vi "LCD Control Panel (No Objects).vi"(8 "error in (no error)":errorcluster) -> (0 "error out":errorcluster)   [LabVIEW 2012]
uses:
  <vilib>/DAQmx/write.llb/DAQmx Write (Analog DBL 1Chan 1Samp).vi
  <vilib>/DAQmx/create/channels.llb/DAQmx Create Channel (AO-Voltage-Basic).vi
  <vilib>/DAQmx/miscellaneous.llb/DAQmx Fill In Error Info.vi
panel:
  out "done":bool
  in  "Analog \nOutput \nSync":bool
  in  "Alternate":bool
  in  "Frequency":dbl=0.01 min=0.01 max=6.0
  out "?":bool
  out "?":bool
  in  "Retardance 2":dbl
  in  "Retardance 1":dbl
  in  "stop":bool
  out "error":bool caption="Error"
  in  "Check for Instrument":bool
  out "Current Retardance":dbl[unit] caption="Retardance"
  out "Ready":bool
  in  "waveoptions":T1(radio) caption="Wave Options"
  in  "Wavelength":dbl[unit]=7.81e-07
  out "Title":string="LCD Retarder Control Program"
  in  "Zero":bool
  in  "Set\nRetardance":bool
  in  "Goto Retardance":dbl[unit]
  in  "Exit":bool
  # "and"
  # "at"
  # "Hz"
  # "between"
  # "Note from John: Analog Output #0 will toggle from 0 to 1 V in synch with this."
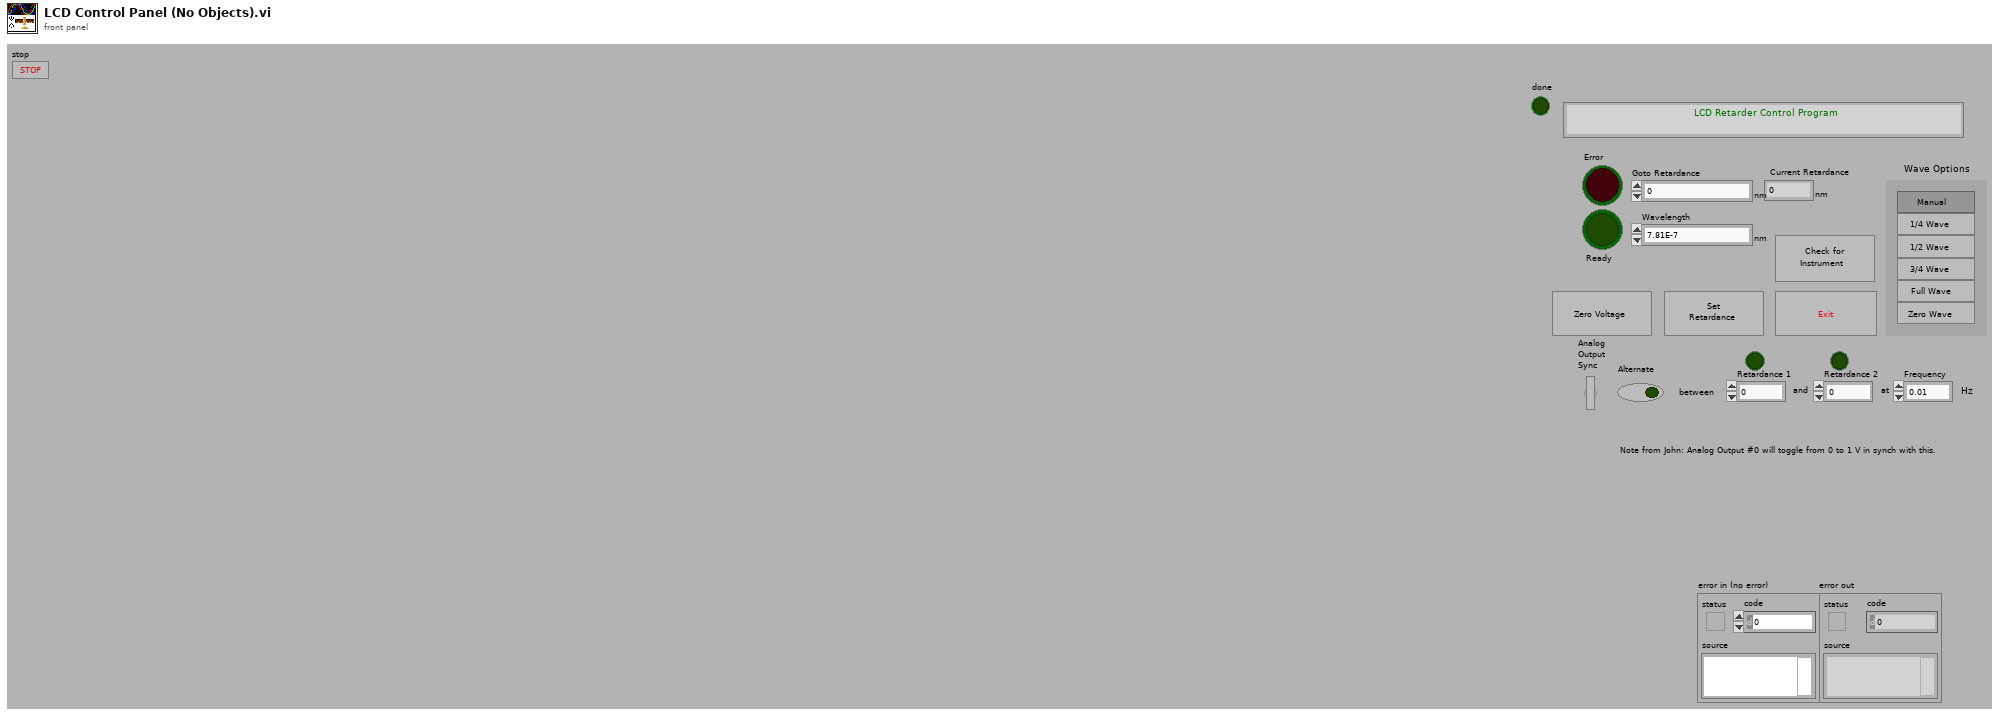
[diagram p1: front panel]
types:
  T1 = enum32{"Manual", "1/4 Wave", "1/2 Wave", "3/4 Wave", "Full Wave", "Zero Wave"}
  T2 = cluster{"Retardance":dbl[unit], "LCD Handle":cluster{"Device Handle":u32, "Pipe 0 Handle":u32, "Pipe 1 Handle":u32}, "All open LCD Handles":cluster{"Device Handle":u32, "Pipe 0 Handle":u32, "Pipe 1 Handle":u32}[], "FW Version":dbl}
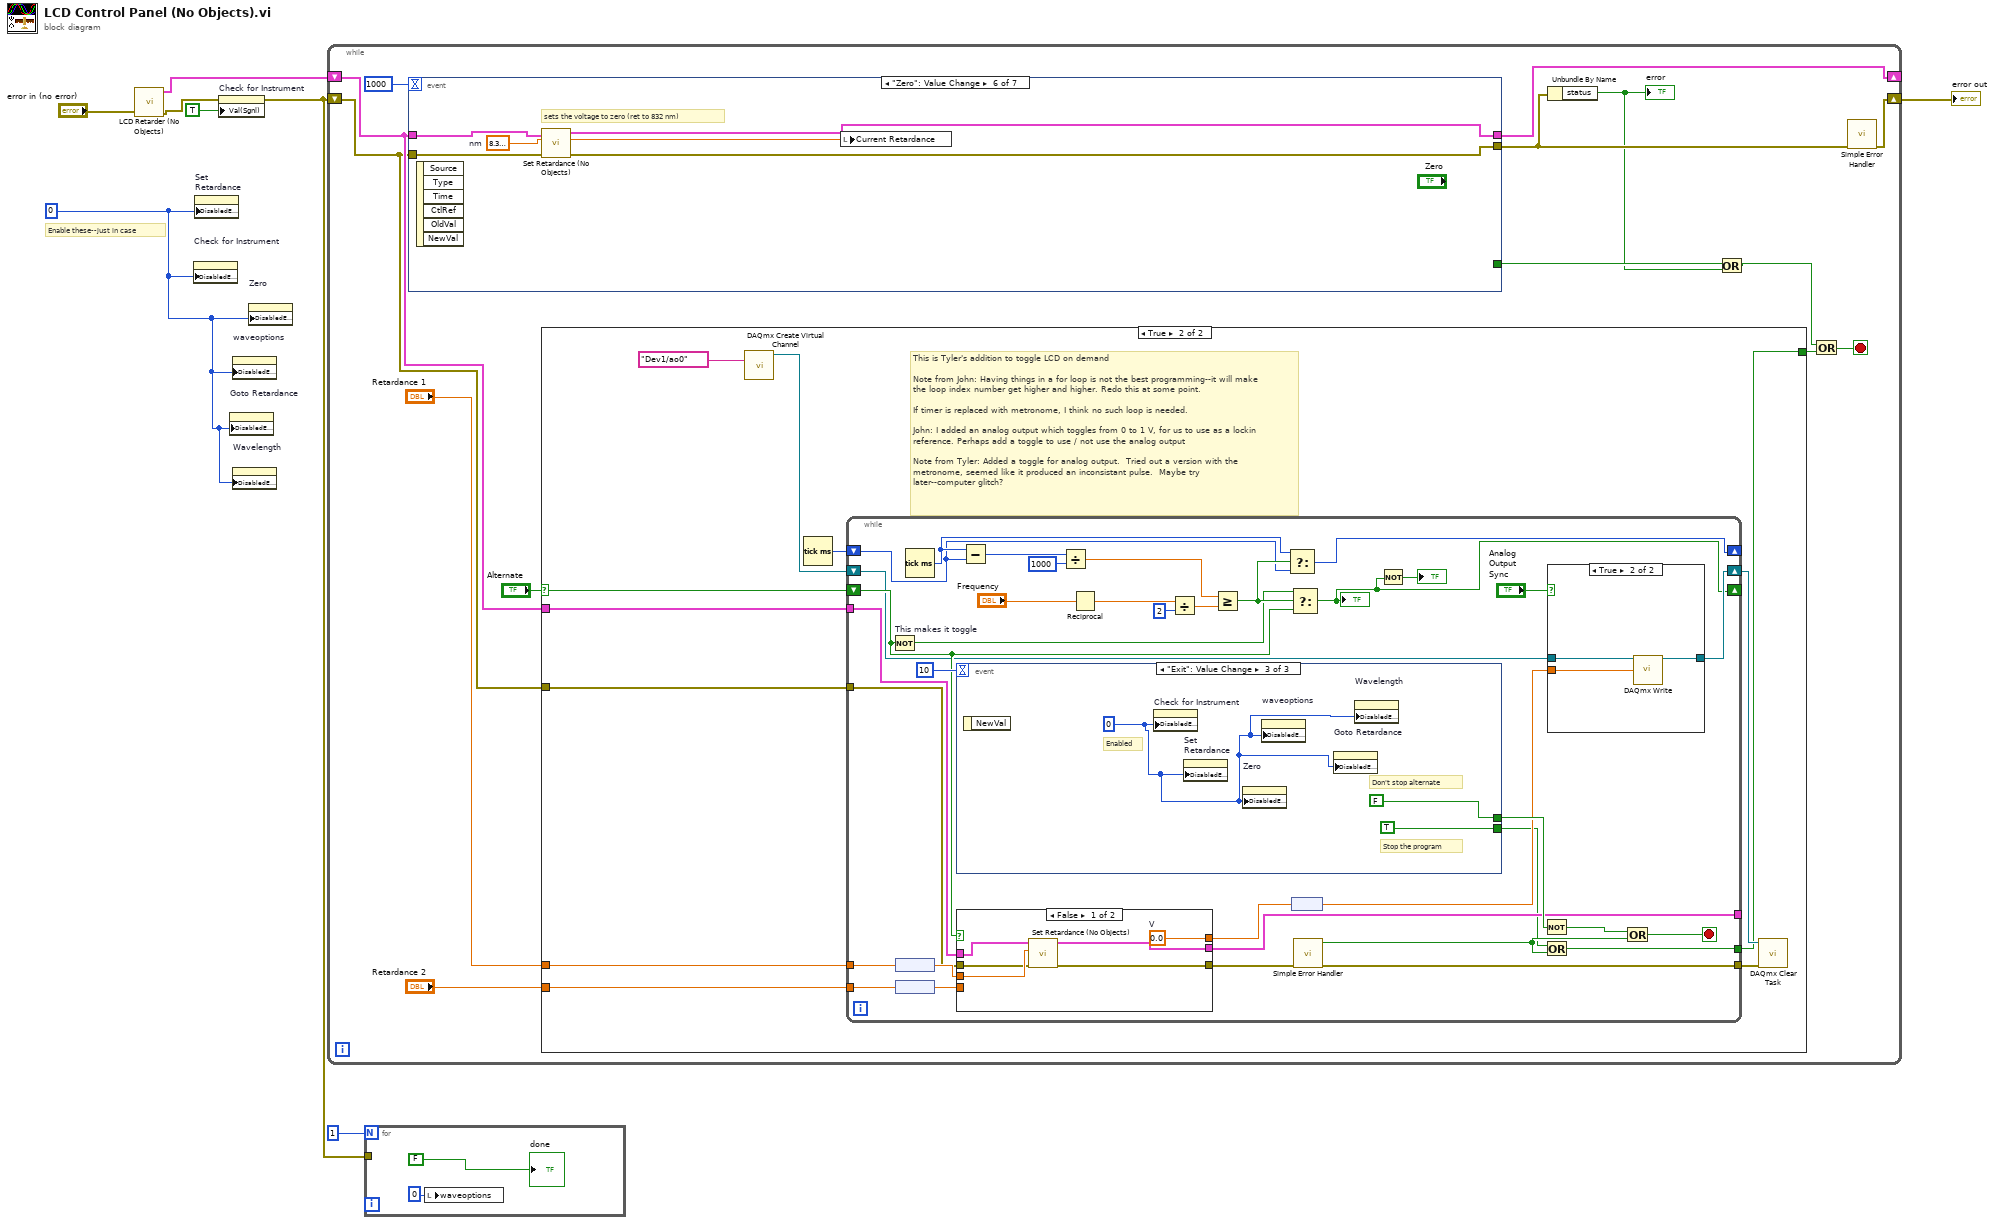
[diagram p0: block diagram]
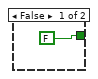
[diagram p2: hidden frame]
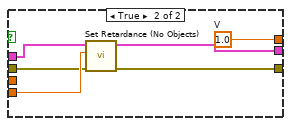
[diagram p4: hidden frame]
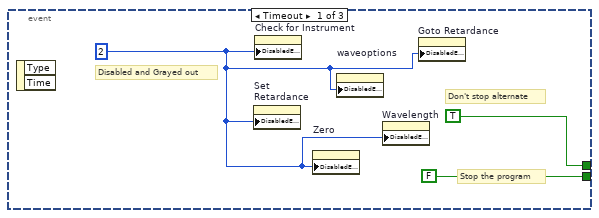
[diagram p5: hidden frame]
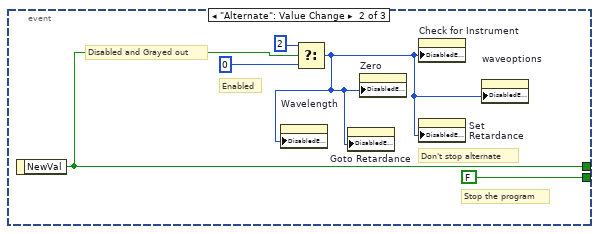
[diagram p6: hidden frame]
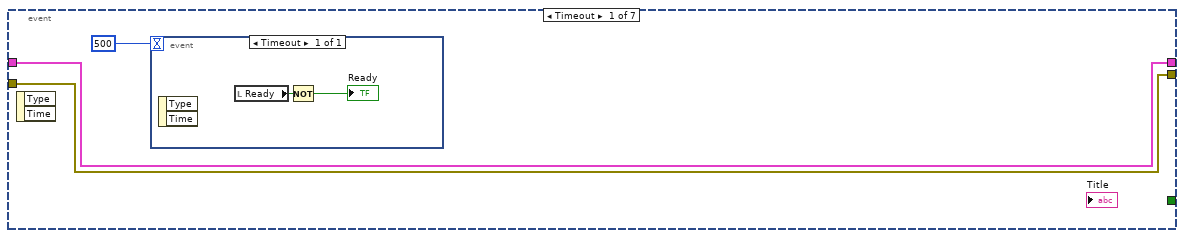
[diagram p7: hidden frame]
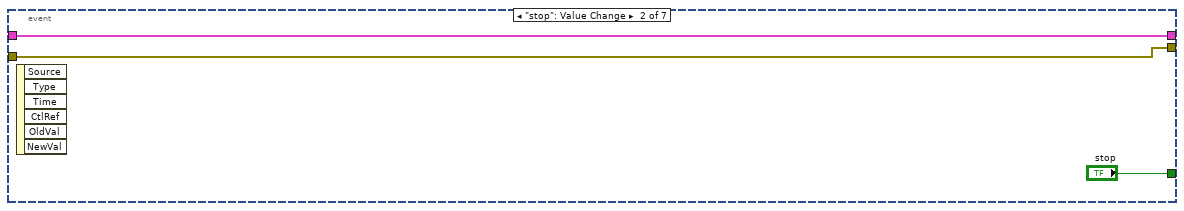
[diagram p8: hidden frame]
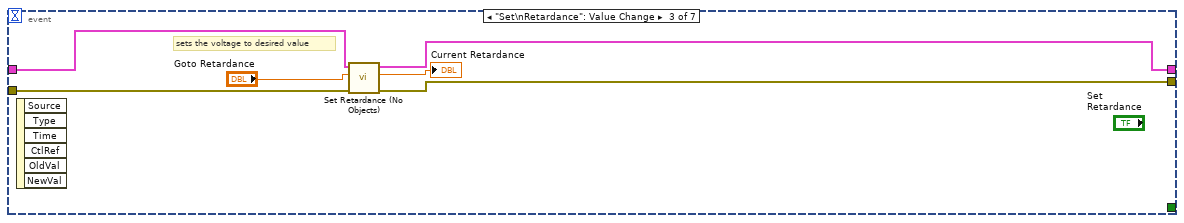
[diagram p9: hidden frame]
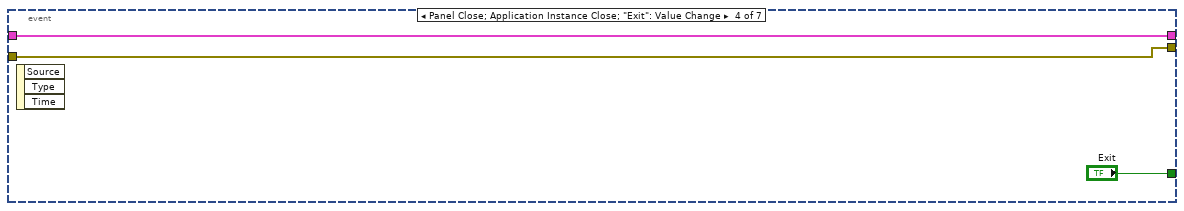
[diagram p10: hidden frame]
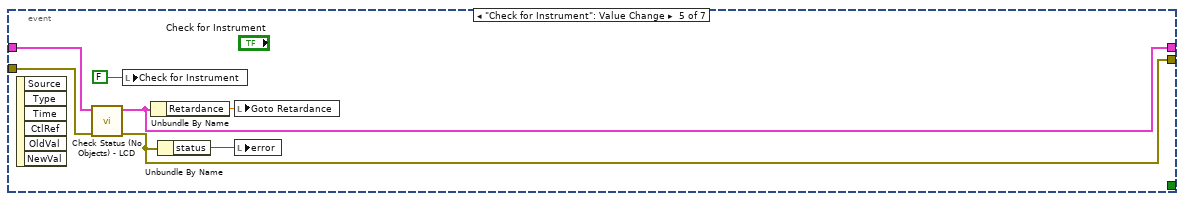
[diagram p11: hidden frame]
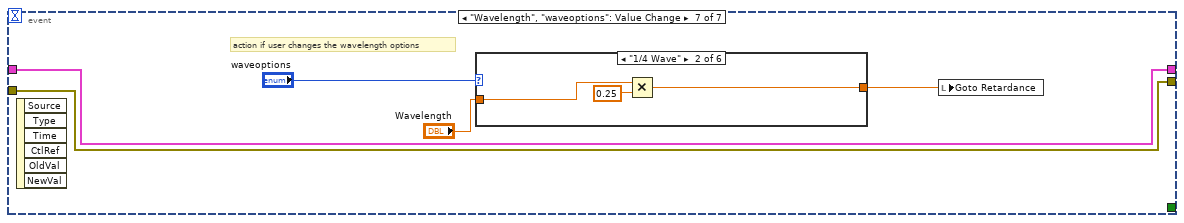
[diagram p12: hidden frame]
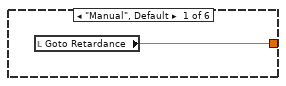
[diagram p13: hidden frame]
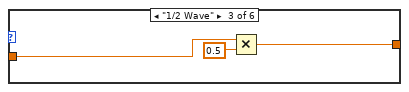
[diagram p14: hidden frame]
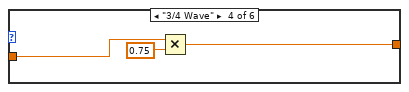
[diagram p15: hidden frame]
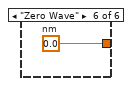
[diagram p17: hidden frame]
diagram:
  w5 = 0
  # "Enable these--just in case"
  n1 = call "LCD Retarder (No Objects).vi"("error in"="error in (no error)") -> ("errorOUT"=w2:errorcluster, "LCD out"=w1:T2)  [unwired: 9 in]
  n2 = property on="Check for Instrument" class="Bool (strict)"("DisabledEnum"=w5) -> ()  [unwired: 2 in, 2 out]
  n3 = property on="Set\nRetardance" class="Bool"("DisabledEnum"=w5) -> ()  [unwired: 2 in, 2 out]
  n4 = property on="Check for Instrument" class="Bool (strict)"(error in=w2, "Val(Sgnl)"=TRUE ("Value (Signaling)")) -> (error out=w6:errorcluster)  [unwired: 1 in, 1 out]
  n5 = property on="Goto Retardance" class="DigNum (strict)"("DisabledEnum"=w5) -> ()  [unwired: 2 in, 2 out]
  n6 = property on="waveoptions" class="RadioBtnsControl (strict)"("DisabledEnum"=w5) -> ()  [unwired: 2 in, 2 out]
  n7 = property on="Wavelength" class="DigNum (strict)"("DisabledEnum"=w5) -> ()  [unwired: 2 in, 2 out]
  n8 = property on="Zero" class="Bool"("DisabledEnum"=w5) -> ()  [unwired: 2 in, 2 out]
  n9 = while {
    shift-right: [w22] -> _
    shift-left: w1 -> [w15]
    shift-right: [w20] -> w4
    shift-left: w6 -> [w14]
    stop <- w13 stop-if-true
    n10 = event shown="[5] \"Zero\": Value Change" {
      selector: _ -> [_ _ _ _ _ _ _]
      dyn-events: _ -> [_ _ _ _ _ _ _]
      timeout: 1000 -> [_ _ _ _ _ _ _]
      tunnel: [_ "stop" _ "Exit" _ _ _] -> w10
      tunnel: [w99 w104 w110 w113 w118 w124 w130] -> w21
      tunnel: w14 -> [w99 w104 w109 w113 w121 w125 w130]
      tunnel: [w100 w103 w111 w114 w115 w123 w131] -> w22
      tunnel: w15 -> [w100 w103 w106 w114 w116 w122 w131]
      event Timeout {
        n11 = event-data() -> ()  [unwired: 3 out]
        n12 = event shown="[0] Timeout" {
          selector: _ -> [_]
          dyn-events: _ -> [_]
          timeout: 500 -> [_]
          event Timeout {
            n13 = event-data() -> ()  [unwired: 1 in, 2 out]
            n14 = local read "Ready"() -> (w102:bool)
            n15 = Not(x=w102) -> (.not. x?=→"Ready":bool)
          }
        }
      }
      event "stop": Value Change {
        n16 = event-data() -> ()  [unwired: 7 out]
      }
      event "Set\nRetardance": Value Change {
        # "sets the voltage to desired value"
        n17 = event-data() -> ()  [unwired: 7 out]
        n18 = call "Set Retardance (No Objects).vi"("errorIN"=w109, "Retardance"="Goto Retardance", "Cluster In"=w106) -> ("errorOUT"=w110:errorcluster, "Retardance out"=→"Current Retardance":dbl[unit], "Cluster Out"=w111:T2)  [unwired: 6 in]
      }
      event Panel Close; Application Instance Close; "Exit": Value Change {
        n19 = event-data() -> ()  [unwired: 4 out]
      }
      event "Check for Instrument": Value Change {
        n20 = event-data() -> ()  [unwired: 7 out]
        n21 = call "Check Status (No Objects) - LCD.vi"("error in (no error)"=w121, "Cluster In"=w116) -> ("error out"=w118:errorcluster, "Cluster Out"=w115:T2)  [unwired: 6 in, 2 out]
        n22 = local write "Check for Instrument"(FALSE ("Check for Instrument")) -> ()
        n23 = Unbundle By Name(w115) -> ("Retardance"=w120:dbl[unit])
        n24 = Unbundle By Name(w118) -> ("status"=w117:bool)
        n25 = local write "Goto Retardance"(w120) -> ()
        n26 = local write "error"(w117) -> ()
      }
      event "Zero": Value Change {
        w126 = dbl[unit] 8.32e-07  # nm
        # "sets the voltage to zero (ret to 832 nm)"
        n27 = event-data() -> ()  [unwired: 7 out]
        n28 = call "Set Retardance (No Objects).vi"("errorIN"=w125, "Retardance"=w126, "Cluster In"=w122) -> ("errorOUT"=w124:errorcluster, "Retardance out"=w127:dbl[unit], "Cluster Out"=w123:T2)  [unwired: 6 in]
        n29 = local write "Current Retardance"(w127) -> ()
      }
      event "Wavelength", "waveoptions": Value Change {
        # "action if user changes the wavelength options"
        n30 = event-data() -> ()  [unwired: 7 out]
        n31 = case shown="\"1/4 Wave\"" "waveoptions" {
          tunnel: "Wavelength" -> [_ w136 w139 w142 w143 _]
          tunnel: [w133 w134 w137 w140 w143 w144] -> w132
          frame "Manual", Default {
            n32 = local read "Goto Retardance"() -> (w133:dbl[unit])
          }
          frame "1/4 Wave" {
            n33 = Multiply(x=w136, y=0.25) -> (x*y=w134:dbl[unit])
          }
          frame "1/2 Wave" {
            n34 = Multiply(x=w139, y=0.5) -> (x*y=w137:dbl[unit])
          }
          frame "3/4 Wave" {
            n35 = Multiply(x=w142, y=0.75) -> (x*y=w140:dbl[unit])
          }
          frame "Full Wave" {
          }
          frame "Zero Wave" {
            w144 = dbl[unit] 0.0  # nm
          }
        }
        n36 = local write "Goto Retardance"(w132) -> ()
      }
    }
    n37 = case shown="True" "Alternate" {
      selector: "Alternate" -> [_ w33]
      tunnel: "Retardance 1" -> [_ w32]
      tunnel: "Retardance 2" -> [_ w31]
      tunnel: w15 -> [_ w26]
      tunnel: w14 -> [_ w25]
      tunnel: [FALSE w24] -> w12
      frame False {
      }
      frame True {
        # "This is Tyler's addition to toggle LCD on demand\n\nNote from John: Having things in a for loop is not the best programming--it will make the loop index number get higher and higher. Redo this at some point.\n\nIf timer is replaced with metronome, I think no such loop is needed.\n\nJohn: I added an analog output which toggles from 0 to 1 V, for us to use as a lockin reference. Perhaps add a toggle to use / not use the analog output\n\nNote from Tyler: Added a toggle for analog output.  Tried out a version with the metronome, seemed like it produced an inconsistant pulse.  Maybe try later--computer glitch?"
        n38 = call-poly <vilib>:"DAQmx Create Virtual Channel.vi"("physical channels"=tag "Dev1/ao0") -> ("task out"=w29:refnum<k21>)  [unwired: 13 in, 1 out]
        n39 = Tick Count (ms)() -> (millisecond timer value=w34:u32)
        n40 = while {
          shift-right: [w58] -> _
          shift-left: w34 -> [w59]
          shift-right: [w46] -> _
          shift-left: w33 -> [w57]
          tunnel: [w56] -> _
          tunnel: [w40] -> w27
          tunnel: w32 -> [w55]
          tunnel: w31 -> [w54]
          tunnel: w26 -> [w52]
          tunnel: w25 -> [w53]
          shift-right: [w49] -> w28
          shift-left: w29 -> [w48]
          tunnel: [w37] -> w24
          stop <- w38 stop-if-true
          n41 = Not "This makes it toggle"(x=w57) -> (.not. x?=w61:bool)
          n42 = node(w55) -> (w68:dbl[unit])
          n43 = node(w54) -> (w67:dbl[unit])
          n44 = Tick Count (ms)() -> (millisecond timer value=w63:u32)
          n45 = event shown="[2] \"Exit\": Value Change" {
            selector: _ -> [_ _ _]
            dyn-events: _ -> [_ _ _]
            timeout: 10 -> [_ _ _]
            tunnel: [TRUE w92 FALSE] -> w69
            tunnel: [FALSE FALSE TRUE] -> w35
            event Timeout {
              w87 = 2
              # "Don't stop alternate"
              # "Stop the program"
              # "Disabled and Grayed out"
              n46 = event-data() -> ()  [unwired: 1 in, 2 out]
              n47 = property on="Set\nRetardance" class="Bool"("DisabledEnum"=w87) -> ()  [unwired: 2 in, 2 out]
              n48 = property on="Check for Instrument" class="Bool (strict)"("DisabledEnum"=w87) -> ()  [unwired: 2 in, 2 out]
              n49 = property on="Zero" class="Bool"("DisabledEnum"=w87) -> ()  [unwired: 2 in, 2 out]
              n50 = property on="waveoptions" class="RadioBtnsControl (strict)"("DisabledEnum"=w87) -> ()  [unwired: 2 in, 2 out]
              n51 = property on="Wavelength" class="DigNum (strict)"("DisabledEnum"=w87) -> ()  [unwired: 2 in, 2 out]
              n52 = property on="Goto Retardance" class="DigNum (strict)"("DisabledEnum"=w87) -> ()  [unwired: 2 in, 2 out]
            }
            event "Alternate": Value Change {
              # "Enabled"
              # "Disabled and Grayed out"
              # "Don't stop alternate"
              # "Stop the program"
              n53 = event-data() -> ("NewVal"=w92:bool)  [unwired: 1 in]
              n54 = Select(t=2, s=w92, f=0) -> (s? t:f=w90:i32)
              n55 = property on="Wavelength" class="DigNum (strict)"("DisabledEnum"=w90) -> ()  [unwired: 2 in, 2 out]
              n56 = property on="Goto Retardance" class="DigNum (strict)"("DisabledEnum"=w90) -> ()  [unwired: 2 in, 2 out]
              n57 = property on="Zero" class="Bool"("DisabledEnum"=w90) -> ()  [unwired: 2 in, 2 out]
              n58 = property on="Check for Instrument" class="Bool (strict)"("DisabledEnum"=w90) -> ()  [unwired: 2 in, 2 out]
              n59 = property on="Set\nRetardance" class="Bool"("DisabledEnum"=w90) -> ()  [unwired: 2 in, 2 out]
              n60 = property on="waveoptions" class="RadioBtnsControl (strict)"("DisabledEnum"=w90) -> ()  [unwired: 2 in, 2 out]
            }
            event "Exit": Value Change {
              w95 = 0
              # "Enabled"
              # "Don't stop alternate"
              # "Stop the program"
              n61 = event-data() -> ()  [unwired: 1 in, 1 out]
              n62 = property on="Check for Instrument" class="Bool (strict)"("DisabledEnum"=w95) -> ()  [unwired: 2 in, 2 out]
              n63 = property on="Set\nRetardance" class="Bool"("DisabledEnum"=w95) -> ()  [unwired: 2 in, 2 out]
              n64 = property on="Zero" class="Bool"("DisabledEnum"=w95) -> ()  [unwired: 2 in, 2 out]
              n65 = property on="waveoptions" class="RadioBtnsControl (strict)"("DisabledEnum"=w95) -> ()  [unwired: 2 in, 2 out]
              n66 = property on="Goto Retardance" class="DigNum (strict)"("DisabledEnum"=w95) -> ()  [unwired: 2 in, 2 out]
              n67 = property on="Wavelength" class="DigNum (strict)"("DisabledEnum"=w95) -> ()  [unwired: 2 in, 2 out]
            }
          }
          n68 = case shown="False" w57 {
            tunnel: w68 -> [w79 _]
            tunnel: [w80 w86] -> w56
            tunnel: [w78 w85] -> w41
            tunnel: w67 -> [_ w84]
            tunnel: w53 -> [w77 w83]
            tunnel: w52 -> [w75 w81]
            tunnel: [w76 w82] -> w50
            frame False {
              w76 = dbl[unit] 0.0  # V
              n69 = call "Set Retardance (No Objects).vi"("errorIN"=w77, "Retardance"=w79, "Cluster In"=w75) -> ("errorOUT"=w78:errorcluster, "Cluster Out"=w80:T2)  [unwired: 6 in, 1 out]
            }
            frame True {
              w82 = dbl[unit] 1.0  # V
              n70 = call "Set Retardance (No Objects).vi"("errorIN"=w83, "Retardance"=w84, "Cluster In"=w81) -> ("errorOUT"=w85:errorcluster, "Cluster Out"=w86:T2)  [unwired: 6 in, 1 out]
            }
          }
          n71 = Subtract(x=w63, y=w59) -> (x-y=w66:u32)
          n72 = Divide(x=w66, y=1000) -> (x/y=w64:dbl)
          n73 = Reciprocal(x="Frequency") -> (1/x=w44:dbl)
          n74 = Divide(x=w44, y=2) -> (x/y=w45:dbl)
          n75 = Greater Or Equal?(x=w64, y=w45) -> (x >= y?=w62:bool)
          n76 = Select(t=w63, s=w62, f=w59) -> (s? t:f=w58:u32)
          n77 = Select(t=w61, s=w62, f=w57) -> (s? t:f=w46:bool)
          "?" <- w46
          n78 = node(w50) -> (w51:dbl)
          n79 = call <vilib>:"Simple Error Handler.vi"("error in (no error)"=w41) -> ("error?"=w36:bool, "error out"=w40:errorcluster)  [unwired: 1 in, 6 out]
          n80 = Not(x=w46) -> (.not. x?=→"?":bool)
          n81 = Not(x=w69) -> (.not. x?=w39:bool)
          n82 = Or(x=w35, y=w36) -> (x .or. y?=w37:bool)
          n83 = case shown="True" "Analog \nOutput \nSync" {
            tunnel: w51 -> [_ w74]
            tunnel: [w71 w73] -> w49
            tunnel: w48 -> [w71 w72]
            frame False {
            }
            frame True {
              n84 = call-poly <vilib>:"DAQmx Write.vi"("task/channels in"=w72, "data"=w74) -> ("task out"=w73:refnum<k21>)  [unwired: 11 in, 2 out]
            }
          }
          n85 = Or(x=w39, y=w36) -> (x .or. y?=w38:bool)
        }
        n86 = call <vilib>:"DAQmx Clear Task.vi"("task in"=w28, "error in"=w27) -> ()  [unwired: 13 in, 1 out]
      }
    }
    n87 = Unbundle By Name(w21) -> ("status"=w9:bool)
    "error" <- w9
    n88 = Or(x=w10, y=w9) -> (x .or. y?=w11:bool)
    n89 = Or(x=w11, y=w12) -> (x .or. y?=w13:bool)
    n90 = call <vilib>:"Simple Error Handler.vi"("error in (no error)"=w21) -> ("error out"=w20:errorcluster)  [unwired: 1 in, 7 out]
  }
  "error out" <- w4
  n91 = for {
    N: 1 -> [_]
    tunnel: w6 -> [_]
    n92 = local write "waveoptions"(0) -> ()
    "done" <- FALSE
  }
